vi "LS330_Main.vi"() -> ()   [LabVIEW 2021]
uses:
  Scale_Cont.ctl
  LS330_Message_Enum.ctl
  LS330_Status_Bundle.ctl
  LS330_LogSelector.ctl
  LS330_Setting_Cluster.ctl
panel:
  in  "Tab Control 4":enum32{"Overview", "History", "Actions"}(tab)
  out "Temp A":dbl caption="Temperature (K)" format="%.2g"
  out "Heater % A":dbl caption="Heater" format="%#_3g%%"
  out "Set Temp A":dbl caption="Current Set Temp (K)" format="%.2g"
  out "Ramp Rate A":dbl caption="Ramp Rate (K/min)" format="%.1g"
  out "Ramp Mode A":bool caption="Ramp Enabled"
  out "Ramp Busy A":bool caption="Ramp Busy"
  out "Heater Mode A":enum16{"Off", "Low", "Medium", "High"}(ring) caption="Heater Mode"
  out "Temp B":dbl caption="Temperature (K)" format="%.2g"
  out "Heater % B":dbl caption="Heater" format="%#_3g%%"
  out "Set Temp B":dbl caption="Current Set Temp (K)" format="%.2g"
  out "Ramp Rate B":dbl caption="Ramp Rate (K/min)" format="%.1g"
  out "Ramp Mode B":bool caption="Ramp Enabled"
  out "Ramp Busy B":bool caption="Ramp Busy"
  out "Heater Mode B":enum16{"Off", "Low", "Medium", "High"}(ring) caption="Heater Mode"
  out "Loop_A LED":bool
  out "Loop_B LED":bool
  out "Loop A Target":dbl caption="Target (K)" format="%.2g"
  out "Loop B Target":dbl caption="Target (K)" format="%.2g"
  in  "E-Stop":bool
  in  "Exit":bool
  out "XY Graph":T1(graph)
  in  "Tab Control 2":enum32{"Heater Options", "Options", "Read-Me!"}(tab)=enum."Read-Me!"
  in  "Tab Control 3":enum32{"Set Point Mode", "Ramp Mode"}(tab)
  in  "Set Temp A 2":dbl caption="Temp Set (K)" min=0.0 max=320.0 step=1.0 format="%.2g"
  in  "Set Range A":enum16{"Off", "Low", "Medium", "High"}(ring) caption="Range Set"
  in  "Set Temp B 2":dbl caption="Temp Set (K)" min=0.0 max=320.0 step=1.0 format="%.2g"
  in  "Set Range B":enum16{"Off", "Low", "Medium", "High"}(ring) caption="Range Set"
  in  "Read Settings":bool
  in  "Send Settings":bool
  in  "Read_A":bool
  in  "Send_A":bool
  in  "Rate_Temp_A":dbl caption="Ramp Rate (K/min)" min=0.0 max=100.0 step=0.1 format="%.1g"
  in  "End_Temp_A":dbl caption="Ramp End (K)" min=0.0 max=325.0 step=0.01 format="%.2g"
  in  "Start_Temp_A":dbl caption="Ramp Start (K)" min=0.0 max=325.0 step=0.01 format="%.2g"
  in  "Start_Temp_B":dbl caption="Ramp Start (K)" min=0.0 max=325.0 step=0.01 format="%.2g"
  in  "End_Temp_B":dbl caption="Ramp End (K)" min=0.0 max=325.0 step=0.01 format="%.2g"
  in  "Rate_Temp_B":dbl caption="Ramp Rate (K/min)" min=0.0 max=100.0 step=0.1 format="%.1g"
  in  "Send_B":bool
  in  "Read_B":bool
  in  "Set Range Ramp A":enum16{"Off", "Low", "Medium", "High"}(ring) caption="Range Set"
  in  "Set Range Ramp B":enum16{"Off", "Low", "Medium", "High"}(ring) caption="Range Set"
  in  "Tab Control":enum32{"Logging Options", "TC Options"}(tab)
  in  "Log Interval (seconds)":dbl=1.0
  in  "Save_Button":bool
  in  "Log File Location":path=path "C:/Users/C1Lab149/Documents/Labview/MDAQ_GUI_Prog/LS330_Main Folder/TempDir"
  in  "Clear_Button":bool
  in  "Chart Y-Axis Auto Scale":T2
  in  "Chart Interval (seconds)":dbl=1.0
  in  "Chart Zoom Width (hours)":dbl=1.0 min=0.01 max=24.0
  in  "Chart Time Width (hours)":dbl=12.0 min=0.01 max=42.0
  in  "Log File Name":string="LogFile_"
  in  "LakeShore VISA ID":refnum<visa-resource-name>="COM3"
  out "Error Panel":errorcluster
  out "HelpFile":string="8-March-22\n****** Read-Me file for LS335 Temperature Controller LabVIEW Program *******\n\nNotes:\n* LOG FILE SETTINGS:\nYou need to select the desired folder only, where you want the log files to be saved in. \nYou may also change the prefix of the saved files.\nThe file will be stored as prefixYYYY_MM_DD.txt (default is Log_YYYY_MM_DD.txt).\nDo this before starting the run.   \nIf you want to change the log settings during a run,\nstop the run, change the settings, and then restart the run.\n\n* AT STARTUP: if the program doesn't see the LS335, make sure that VISA ID is set to COM9 under the OPTIONS TAB.\n\n* FOR RAMPING: first set and achieve the initial temperature you want to start a ramp from.\n\tThen input the desired temperature you want to ramp to, set the ramp rate, and then enable the 'Toggle Ramping' slider before pressing the 'Send Settings' button.\n\tBoth the 'Ramp Enabled' and 'Ramp Busy' lights should be on and indicates that the LS335 is ramping to your desired temperature. NOTE: The 'Set Temp' indicator shows the steps towards the 'Target' temperature.\n\t\n\tOnce the 'Ramp' busy lights are off, the LS335 has finished the ramp procedure.\n\tYou may then either switch of the ramp slider which would revert the LS335 to the usual behaviour, or input a new set-point with the ramp slider still on. This will cause another ramp to occur.\n\n\tIf 'Send Settings' is pressed again with the 'Toggle Ramping' switch enabled, the ramp target is adjusted to the new value.\n\t\n\n"
  # "Loop A"
  # "Loop B"
  # "Heater A"
  # "Heater B"
  # "Heater A"
  # "Heater B"
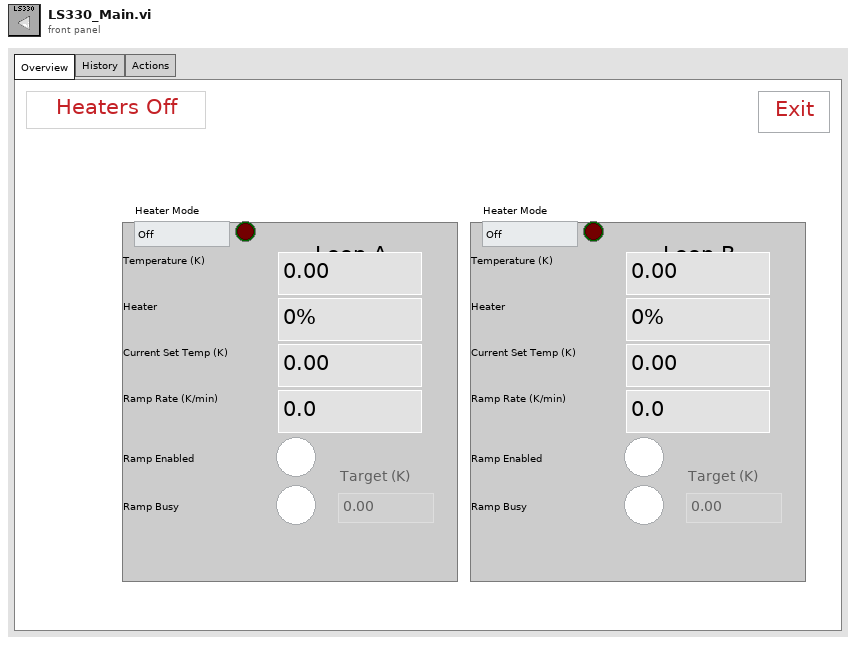
[diagram p1: front panel]
types:
  T1 = cluster{"Array":cluster{"time stamp":timestamp, "Numeric":dbl}[]}[]
  T2 = typedef "Scale_Cont.ctl" = enum16{"A & B", "A", "B"}
  T3 = typedef "LS330_LogSelector.ctl" = enum16{"NewFile", "Log", "OpenFile"}
  T4 = typedef "LS330_Status_Bundle.ctl" = cluster{"Temp":dbl, "Heater %":dbl, "Range":enum16{"Off", "Low", "Medium", "High"}, "Set Temp (K)":dbl, "Ramp Value":dbl, "Ramp Mode On/Off":bool, "Ramp Busy On/Off":bool}
  T5 = typedef "LS330_Message_Enum.ctl" = enum16{"Send Ramp B", "Send Ramp A", "Ramp Read Init B", "Ramp Read Init A", "Monitor TC", "Write Settings", "Read Settings", "E-Stop Write", "Quit Program"}
  T6 = cluster{cluster{timestamp, bool}, "Status IN":cluster{T4, T4}}
  T7 = cluster{"Array":cluster{"time stamp":timestamp, "Numeric":dbl}[], "Array":cluster{"time stamp":timestamp, "Numeric":dbl}[], "Array":cluster{"time stamp":timestamp, "Numeric":dbl}[], "Array":cluster{"time stamp":timestamp, "Numeric":dbl}[]}
  T8 = cluster{"Cluster":cluster{timestamp, "Checkbox":bool}, "Status IN":cluster{T4, T4}}
  T9 = cluster{"Array":cluster{timestamp, "Temp":dbl}[], "Array":cluster{timestamp, "Heater %":dbl}[], "Array":cluster{timestamp, "Temp":dbl}[], "Array":cluster{timestamp, "Heater %":dbl}[]}
  T10 = cluster{"Array":cluster{timestamp, "Heater %":dbl}[]}[]
  T11 = cluster{"TempA_Max":dbl, "TempA_Min":dbl, "HeaterA_Max":dbl, "HeaterA_Min":dbl, "TempB_Max":dbl, "TempB_Min":dbl, "HeaterB_Max":dbl, "HeaterB_Min":dbl}
  T12 = enum8{"Enabled", "Disabled", "Disabled and Grayed Out"}
  T13 = cluster{"seconds since 1Jan1904":timestamp, bool}
  T14 = cluster{cluster{"seconds since 1Jan1904":timestamp, bool}, "Status":cluster{T4, T4}}
  T15 = typedef "LS330_Setting_Cluster.ctl" = cluster{"Set Temp":dbl, "Set Range":enum16{"Off", "Low", "Medium", "High"}, "Set Ramp Rate":dbl, "Toggle Ramping":bool}
  T16 = cluster{"Setting Cluster":T15, "Setting Cluster":T15}
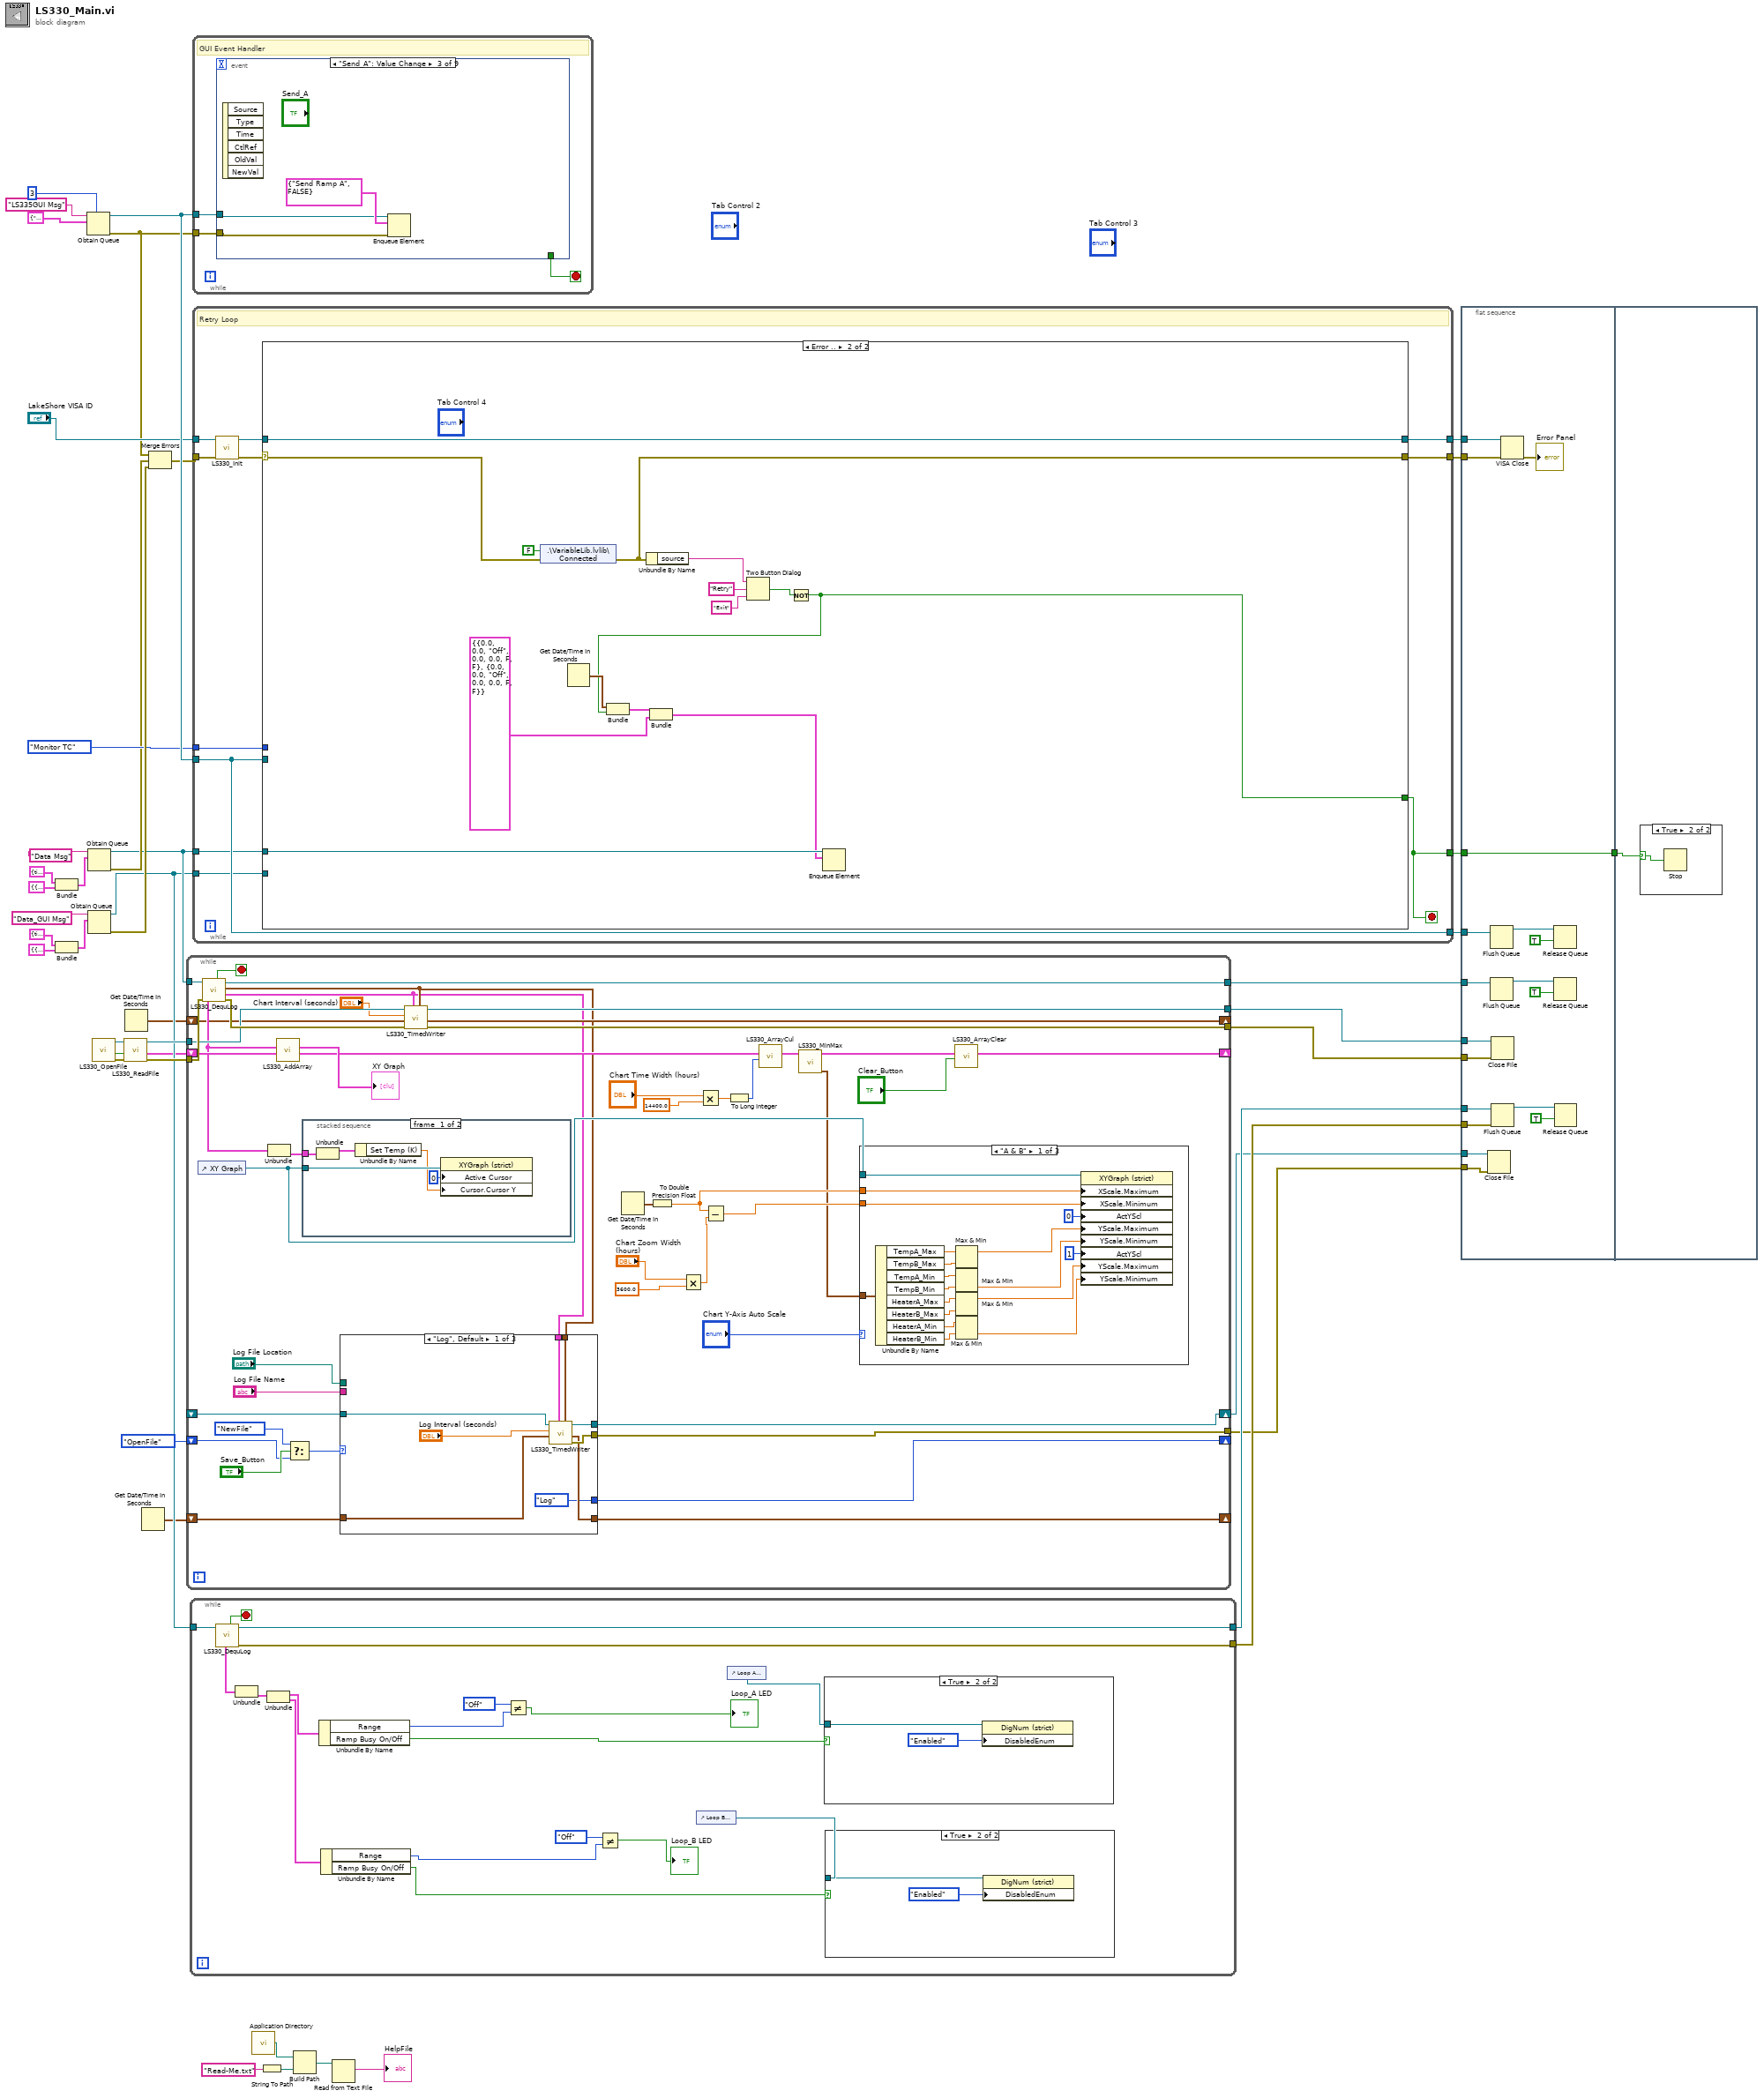
[diagram p0: block diagram]
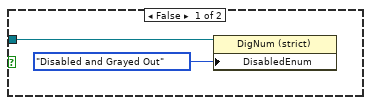
[diagram p2: hidden frame]
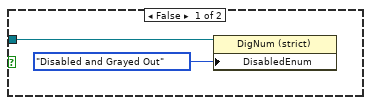
[diagram p3: hidden frame]
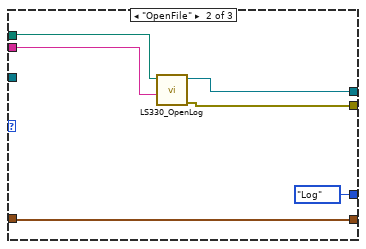
[diagram p4: hidden frame]
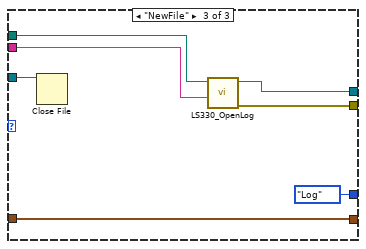
[diagram p5: hidden frame]
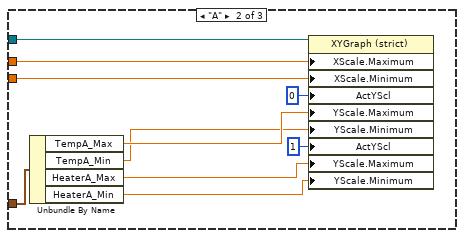
[diagram p6: hidden frame]
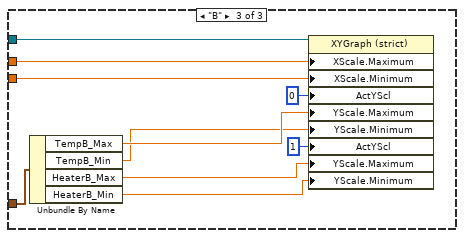
[diagram p7: hidden frame]
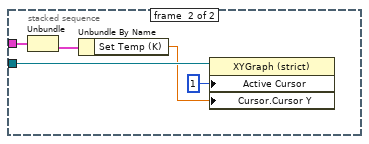
[diagram p8: hidden frame]
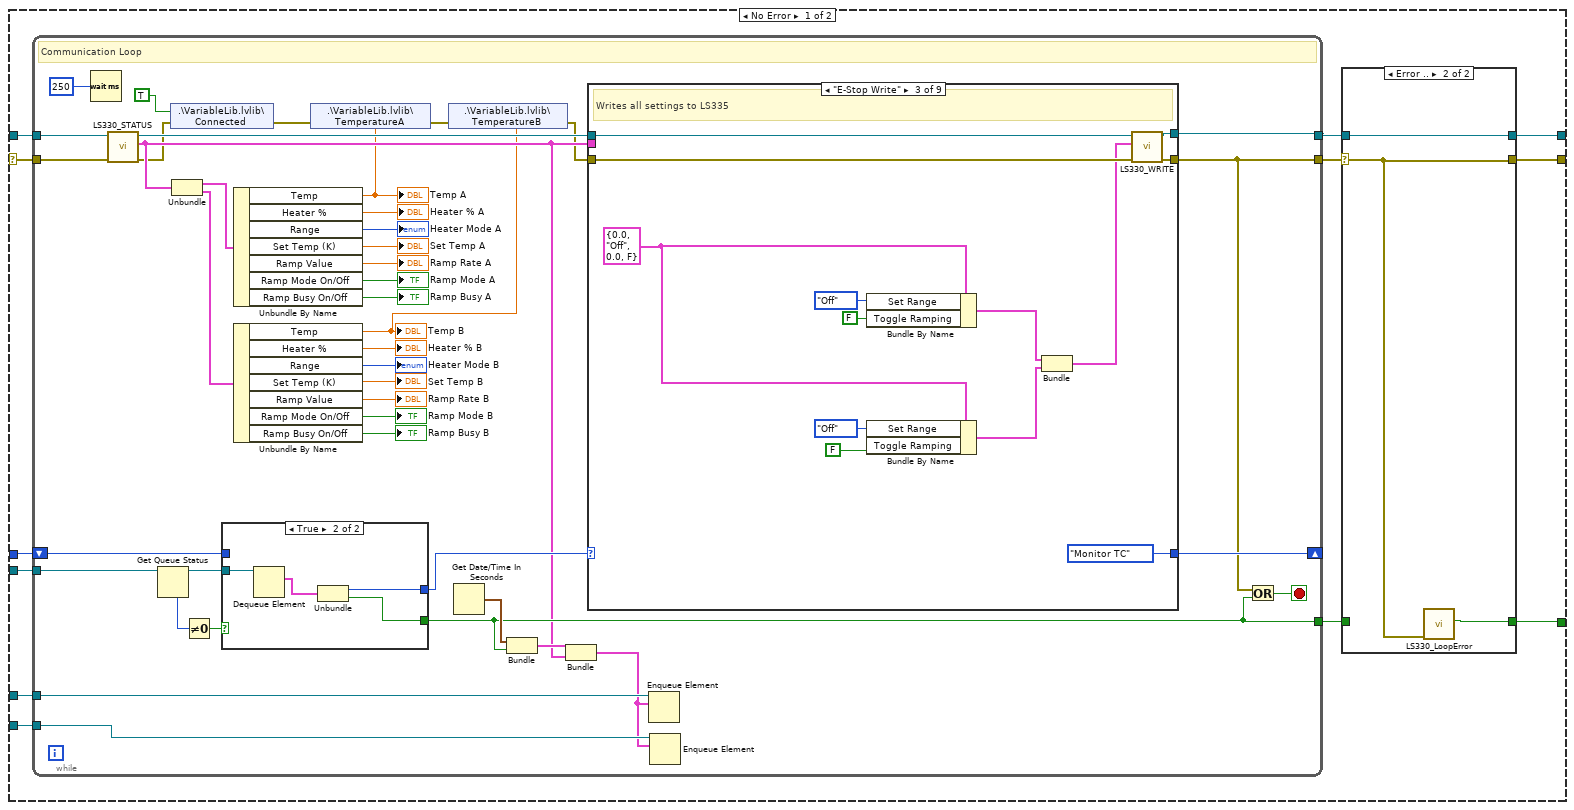
[diagram p10: hidden frame]
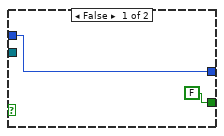
[diagram p12: hidden frame]
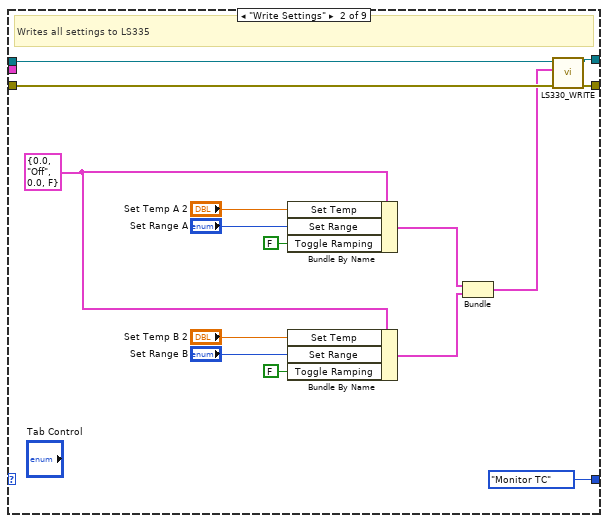
[diagram p14: hidden frame]
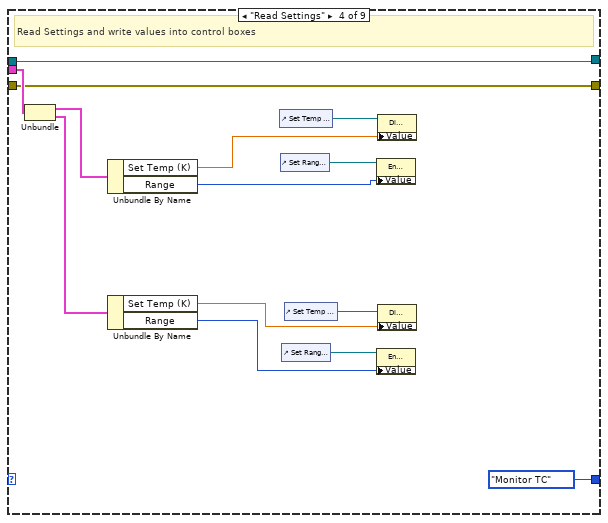
[diagram p15: hidden frame]
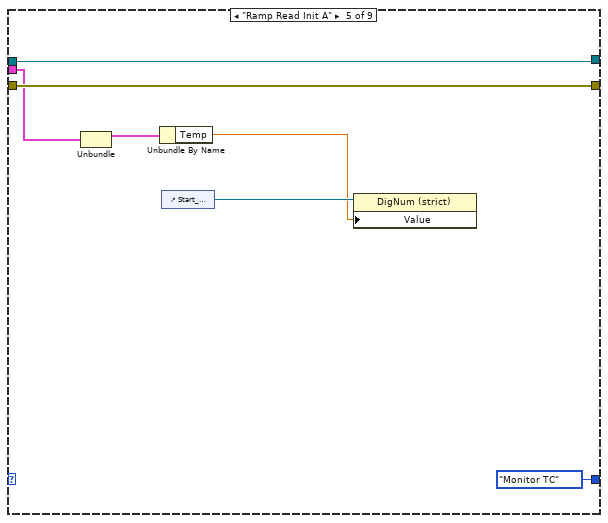
[diagram p16: hidden frame]
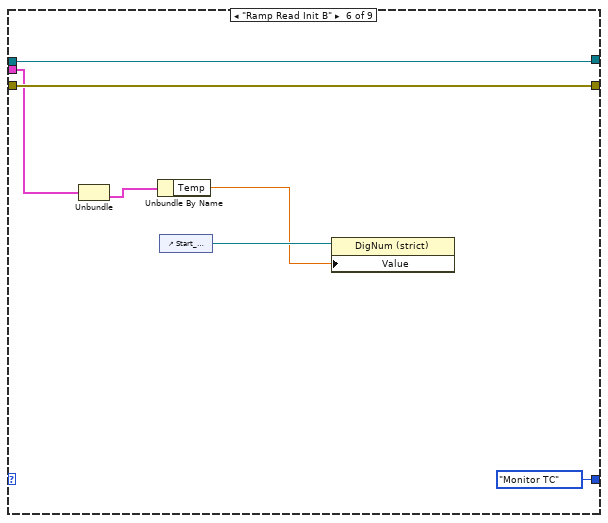
[diagram p17: hidden frame]
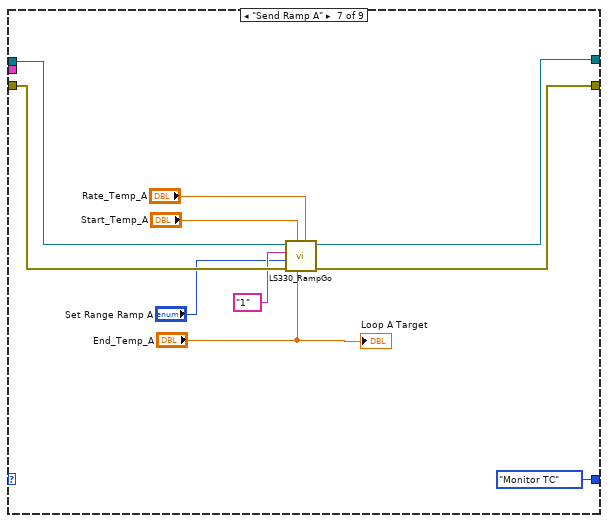
[diagram p18: hidden frame]
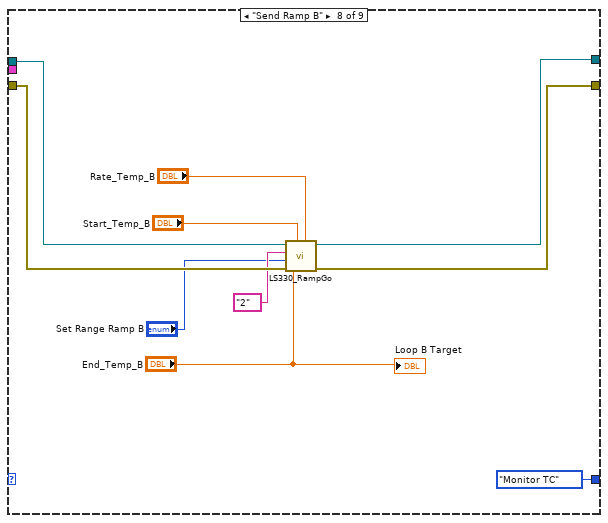
[diagram p19: hidden frame]
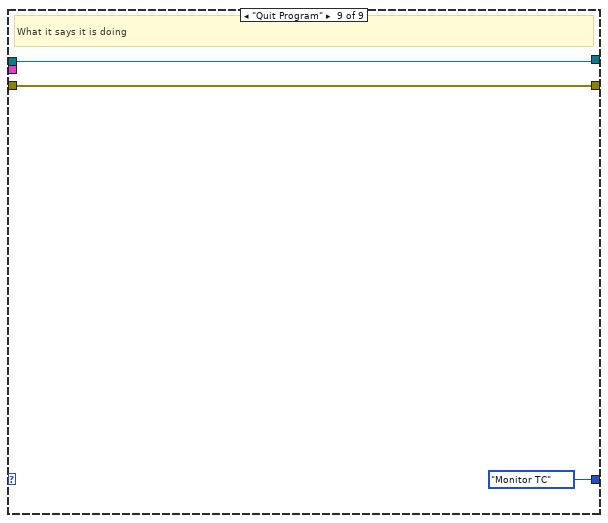
[diagram p20: hidden frame]
diagram:
  n1 = Bundle(cluster{timestamp, bool} {timestamp(0 s since 1904-01-01), FALSE}, "Status IN"=cluster{T4, T4} {{"Temp"=0.0, "Heater %"=0.0, "Range"=enum."Off", "Set Temp (K)"=0.0, "Ramp Value"=0.0, "Ramp Mode On/Off"=FALSE, "Ramp Busy On/Off"=FALSE}, {"Temp"=0.0, "Heater %"=0.0, "Range"=enum."Off", "Set Temp (K)"=0.0, "Ramp Value"=0.0, "Ramp Mode On/Off"=FALSE, "Ramp Busy On/Off"=FALSE}}) -> (w26:T6)  [unwired: 1 in]
  n2 = Bundle(cluster{timestamp, bool} {timestamp(0 s since 1904-01-01), FALSE}, "Status IN"=cluster{T4, T4} {{"Temp"=0.0, "Heater %"=0.0, "Range"=enum."Off", "Set Temp (K)"=0.0, "Ramp Value"=0.0, "Ramp Mode On/Off"=FALSE, "Ramp Busy On/Off"=FALSE}, {"Temp"=0.0, "Heater %"=0.0, "Range"=enum."Off", "Set Temp (K)"=0.0, "Ramp Value"=0.0, "Ramp Mode On/Off"=FALSE, "Ramp Busy On/Off"=FALSE}}) -> (w16:T6)  [unwired: 1 in]
  n3 = Obtain Queue(max queue size (-1, unlimited)=3, name (unnamed)="LS335GUI Msg", element data type=cluster{T5, bool} {enum."Monitor TC", TRUE}) -> (queue out=w45:refnum<queue>, error out=w32:errorcluster)  [unwired: 2 in, 1 out]
  n4 = Obtain Queue(name (unnamed)="Data Msg", element data type=w26) -> (queue out=w30:refnum<queue>, error out=w33:errorcluster)  [unwired: 3 in, 1 out]
  n5 = Obtain Queue(name (unnamed)="Data_GUI Msg", element data type=w16) -> (queue out=w21:refnum<queue>, error out=w46:errorcluster)  [unwired: 3 in, 1 out]
  n6 = call "LS330_OpenFile.vi"() -> ("error out"=w4:errorcluster, "file or folder exists?"=w5:bool, "File RefOut"=w6:refnum<file>)  [unwired: 9 in]
  n7 = call "LS330_ReadFile.vi"("error in"=w4, "File Exists?"=w5, "refnum"=w6) -> ("error out"=w28:errorcluster, "Cluster"=w20:T7, "refnum out"=w29:refnum<file>)  [unwired: 6 in]
  n8 = Get Date/Time In Seconds() -> (seconds since 1Jan1904=w19:timestamp)
  n9 = Get Date/Time In Seconds() -> (seconds since 1Jan1904=w3:timestamp)
  n10 = Merge Errors(w32, w33, w46) -> (w31:errorcluster)
  n11 = while {
    tunnel: w30 -> [w91]
    tunnel: w29 -> [w89]
    tunnel: w28 -> [w93]
    shift-right: [w62] -> _
    shift-left: w20 -> [w88]
    tunnel: [w90] -> w24
    tunnel: [w87] -> w23
    tunnel: [w86] -> w22
    shift-right: [w80] -> _
    shift-left: w19 -> [w81]
    shift-right: [w49] -> _
    shift-left: LS330_LogSelector."OpenFile" -> [w59]
    shift-right: [w51] -> _
    shift-left: w3 -> [w53]
    tunnel: [w52] -> w1
    shift-right: [w50] -> w2
    shift-left: _ -> [w56]
    stop <- w84 stop-if-true
    n12 = control-ref of="XY Graph"() -> (w78:refnum<vi>)
    n13 = call "LS330_DequLog.vi"("error in"=w93, "Queue in"=w91) -> ("error out"=w92:errorcluster, "Status Out"=w54:cluster{T4, T4}, "Time Stamp"=w55:timestamp, "Queue out"=w90:refnum<queue>, "Terminate?"=w84:bool, "Status/Time  Out"=w82:T8)  [unwired: 4 in]
    n14 = Unbundle(w82) -> ("Status IN"=w83:cluster{T4, T4})  [unwired: 1 out]
    n15 = call "LS330_AddArray.vi"("Array Cluster IN"=w88, "Queue IN"=w82) -> ("Array Cluster OUT"=w71:T9, "XY Plot Data"=→"XY Graph":T10)  [unwired: 8 in]
    n16 = Select(t=LS330_LogSelector."NewFile", s="Save_Button", f=w59) -> (s? t:f=w57:T3)
    n17 = stacked-sequence {
      tunnel: w78 -> [w158 w163]
      tunnel: w83 -> [w157 w162]
      frame #0 {
        n18 = Unbundle(w157) -> (w156:T4)  [unwired: 1 out]
        n19 = Unbundle By Name(w156) -> ("Set Temp (K)"=w155:dbl)
        n20 = property class="XYGraph (strict)"(reference=w158, "Active Cursor"=u32 0, "Cursor.Cursor Y"=w155) -> ()  [unwired: 1 in, 2 out]
      }
      frame #1 {
        n21 = Unbundle(w162) -> (w160:T4)  [unwired: 1 out]
        n22 = Unbundle By Name(w160) -> ("Set Temp (K)"=w161:dbl)
        n23 = property class="XYGraph (strict)"(reference=w163, "Active Cursor"=u32 1, "Cursor.Cursor Y"=w161) -> ()  [unwired: 1 in, 2 out]
      }
    }
    n24 = case shown="\"Log\", Default" w57 {
      tunnel: w56 -> [w94 _ w115]
      tunnel: w55 -> [w102 _ _]
      tunnel: w54 -> [w101 _ _]
      tunnel: w53 -> [w100 w105 w110]
      tunnel: [w99 w107 w111] -> w52
      tunnel: [w98 w105 w110] -> w51
      tunnel: [w97 w108 w112] -> w50
      tunnel: [LS330_LogSelector."Log" ("t") LS330_LogSelector."Log" ("t") LS330_LogSelector."Log" ("t")] -> w49
      tunnel: "Log File Name" -> [_ w104 w113]
      tunnel: "Log File Location" -> [_ w103 w114]
      frame "Log", Default {
        n25 = call "LS330_TimedWriter.vi"("Time Stamp"=w102, "Status In"=w101, "Time Check In"=w100, "Interval"="Log Interval (seconds)", "Byte Stream File in"=w94) -> ("error out"=w99:errorcluster, "Time Check Out"=w98:timestamp, "Byte Stream File out"=w97:refnum<file>)  [unwired: 4 in]
      }
      frame "OpenFile" {
        n26 = call "LS330_OpenLog.vi"("Prefix"=w104, "Log Location"=w103) -> ("error out"=w107:errorcluster, "File RefOut"=w108:refnum<file>)  [unwired: 7 in, 1 out]
      }
      frame "NewFile" {
        n27 = Close File(refnum=w115) -> ()  [unwired: 1 in, 2 out]
        n28 = call "LS330_OpenLog.vi"("Prefix"=w113, "Log Location"=w114) -> ("error out"=w111:errorcluster, "File RefOut"=w112:refnum<file>)  [unwired: 7 in, 1 out]
      }
    }
    n29 = call "LS330_TimedWriter.vi"("Time Stamp"=w55, "Status In"=w54, "error in (no error)"=w92, "Time Check In"=w81, "Interval"="Chart Interval (seconds)", "Byte Stream File in"=w89) -> ("error out"=w86:errorcluster, "Time Check Out"=w80:timestamp, "Byte Stream File out"=w87:refnum<file>)  [unwired: 3 in]
    n30 = Get Date/Time In Seconds() -> (seconds since 1Jan1904=w77:timestamp)
    n31 = To Double Precision Float(number=w77) -> (double precision float=w76:dbl)
    n32 = Multiply(x="Chart Zoom Width (hours)", y=3600.0) -> (x*y=w73:dbl)
    n33 = Multiply(x="Chart Time Width (hours)", y=14400.0) -> (x*y=w68:dbl)
    n34 = Subtract(x=w76, y=w73) -> (x-y=w72:dbl)
    n35 = To Long Integer(number=w68) -> (32bit integer=w67:i32)
    n36 = call "LS330_ArrayCul.vi"("Max Size"=w67, "Cluster Array IN"=w71) -> ("output cluster"=w66:T7)  [unwired: 9 in]
    n37 = call "LS330_MinMax.vi"("Input Cluster"=w66) -> ("Value Cluster"=w64:T11, "output cluster"=w63:T7)  [unwired: 9 in]
    n38 = case shown="\"A & B\"" "Chart Y-Axis Auto Scale" {
      tunnel: w78 -> [w133 w143 w153]
      tunnel: w76 -> [w132 w142 w152]
      tunnel: w72 -> [w131 w141 w151]
      tunnel: w64 -> [w130 w140 w150]
      frame "A & B" {
        n39 = Unbundle By Name(w130) -> ("TempA_Max"=w129:dbl, "TempB_Max"=w128:dbl, "TempA_Min"=w125:dbl, "TempB_Min"=w124:dbl, "HeaterA_Max"=w121:dbl, "HeaterB_Max"=w120:dbl, "HeaterA_Min"=w118:dbl, "HeaterB_Min"=w117:dbl)
        n40 = Max & Min(x=w129, y=w128) -> (max(x,y)=w126:dbl)  [unwired: 1 out]
        n41 = Max & Min(x=w125, y=w124) -> (min(x,y)=w123:dbl)  [unwired: 1 out]
        n42 = Max & Min(x=w121, y=w120) -> (max(x,y)=w119:dbl)  [unwired: 1 out]
        n43 = Max & Min(x=w118, y=w117) -> (min(x,y)=w116:dbl)  [unwired: 1 out]
        n44 = property class="XYGraph (strict)"(reference=w133, "XScale.Maximum"=w132, "XScale.Minimum"=w131, "ActYScl"=0 ("Active Y Scale"), "YScale.Maximum"=w126, "YScale.Minimum"=w123, "ActYScl"=1 ("Active Y Scale"), "YScale.Maximum"=w119, "YScale.Minimum"=w116) -> ()  [unwired: 1 in, 2 out]
      }
      frame "A" {
        n45 = Unbundle By Name(w140) -> ("TempA_Max"=w137:dbl, "TempA_Min"=w136:dbl, "HeaterA_Max"=w135:dbl, "HeaterA_Min"=w134:dbl)
        n46 = property class="XYGraph (strict)"(reference=w143, "XScale.Maximum"=w142, "XScale.Minimum"=w141, "ActYScl"=0 ("Active Y Scale"), "YScale.Maximum"=w137, "YScale.Minimum"=w136, "ActYScl"=1 ("Active Y Scale"), "YScale.Maximum"=w135, "YScale.Minimum"=w134) -> ()  [unwired: 1 in, 2 out]
      }
      frame "B" {
        n47 = Unbundle By Name(w150) -> ("TempB_Max"=w147:dbl, "TempB_Min"=w146:dbl, "HeaterB_Max"=w145:dbl, "HeaterB_Min"=w144:dbl)
        n48 = property class="XYGraph (strict)"(reference=w153, "XScale.Maximum"=w152, "XScale.Minimum"=w151, "ActYScl"=0 ("Active Y Scale"), "YScale.Maximum"=w147, "YScale.Minimum"=w146, "ActYScl"=1 ("Active Y Scale"), "YScale.Maximum"=w145, "YScale.Minimum"=w144) -> ()  [unwired: 1 in, 2 out]
      }
    }
    n49 = call "LS330_ArrayClear.vi"("Clear"="Clear_Button", "input cluster"=w63) -> ("output cluster"=w62:T7)  [unwired: 9 in]
  }
  n50 = while {
    tunnel: w21 -> [w181]
    tunnel: [w164] -> w14
    tunnel: [w179] -> w13
    stop <- w180 stop-if-true
    n51 = call "LS330_DequLog.vi"("Queue in"=w181) -> ("error out"=w179:errorcluster, "Queue out"=w164:refnum<queue>, "Terminate?"=w180:bool, "Status/Time  Out"=w178:T8)  [unwired: 5 in, 2 out]
    n52 = Unbundle(w178) -> ("Status IN"=w177:cluster{T4, T4})  [unwired: 1 out]
    n53 = Unbundle(w177) -> (w176:T4, w175:T4)
    n54 = Unbundle By Name(w176) -> ("Range"=w174:enum16{"Off", "Low", "Medium", "High"}, "Ramp Busy On/Off"=w168:bool)
    n55 = Unbundle By Name(w175) -> ("Range"=w170:enum16{"Off", "Low", "Medium", "High"}, "Ramp Busy On/Off"=w165:bool)
    n56 = Not Equal?(x=enum16{"Off", "Low", "Medium", "High"}."Off", y=w174) -> (x != y?=→"Loop_A LED":bool)
    n57 = Not Equal?(x=enum16{"Off", "Low", "Medium", "High"}."Off", y=w170) -> (x != y?=→"Loop_B LED":bool)
    n58 = control-ref of="Loop B Target"() -> (w166:refnum<vi>)
    n59 = control-ref of="Loop A Target"() -> (w167:refnum<vi>)
    n60 = case shown="True" w168 {
      tunnel: w167 -> [w187 w189]
      frame False {
        n61 = property class="DigNum (strict)"(reference=w187, "DisabledEnum"=T12."Disabled and Grayed Out" ("Disabled")) -> ()  [unwired: 1 in, 2 out]
      }
      frame True {
        n62 = property class="DigNum (strict)"(reference=w189, "DisabledEnum"=T12."Enabled" ("Disabled")) -> ()  [unwired: 1 in, 2 out]
      }
    }
    n63 = case shown="True" w165 {
      tunnel: w166 -> [w183 w185]
      frame False {
        n64 = property class="DigNum (strict)"(reference=w183, "DisabledEnum"=T12."Disabled and Grayed Out" ("Disabled")) -> ()  [unwired: 1 in, 2 out]
      }
      frame True {
        n65 = property class="DigNum (strict)"(reference=w185, "DisabledEnum"=T12."Enabled" ("Disabled")) -> ()  [unwired: 1 in, 2 out]
      }
    }
  }
  n66 = while "GUI Event Handler" {
    tunnel: w45 -> [w192]
    tunnel: w32 -> [w191]
    stop <- w190 stop-if-true
    # "GUI Event Handler"
    n67 = event shown="[2] \"Send_A\": Value Change" {
      selector: _ -> [_ _ _ _ _ _ _ _ _]
      dyn-events: _ -> [_ _ _ _ _ _ _ _ _]
      timeout: _ -> [_ _ _ _ _ _ _ _ _]
      tunnel: w192 -> [_ w195 w198 w201 w204 w207 w211 w216 w220]
      tunnel: w191 -> [_ w194 w197 w200 w203 w206 w209 w214 w219]
      tunnel: [_ FALSE _ _ _ _ FALSE TRUE FALSE] -> w190
      event Timeout {
        n68 = event-data() -> ()  [unwired: 1 in, 3 out]
      }
      event "Send Settings": Value Change {
        n69 = event-data() -> ()  [unwired: 1 in, 6 out]
        n70 = Enqueue Element(queue=w195, element=cluster{T5, bool} {enum."Write Settings", FALSE}, error in (no error)=w194) -> ()  [unwired: 1 in, 3 out]
      }
      event "Send_A": Value Change {
        n71 = event-data() -> ()  [unwired: 1 in, 6 out]
        n72 = Enqueue Element(queue=w198, element=cluster{T5, bool} {enum."Send Ramp A", FALSE}, error in (no error)=w197) -> ()  [unwired: 1 in, 3 out]
      }
      event "Send_B": Value Change {
        n73 = event-data() -> ()  [unwired: 1 in, 6 out]
        n74 = Enqueue Element(queue=w201, element=cluster{T5, bool} {enum."Send Ramp B", FALSE}, error in (no error)=w200) -> ()  [unwired: 1 in, 3 out]
      }
      event "Read_A": Value Change {
        n75 = event-data() -> ()  [unwired: 1 in, 6 out]
        n76 = Enqueue Element(queue=w204, element=cluster{T5, bool} {enum."Ramp Read Init A", FALSE}, error in (no error)=w203) -> ()  [unwired: 1 in, 3 out]
      }
      event "Read_B": Value Change {
        n77 = event-data() -> ()  [unwired: 1 in, 6 out]
        n78 = Enqueue Element(queue=w207, element=cluster{T5, bool} {enum."Ramp Read Init B", FALSE}, error in (no error)=w206) -> ()  [unwired: 1 in, 3 out]
      }
      event "Read Settings": Value Change {
        n79 = event-data() -> ()  [unwired: 1 in, 6 out]
        n80 = Enqueue Element(queue=w211, element=cluster{T5, bool} {enum."Read Settings", FALSE}, error in (no error)=w209) -> ()  [unwired: 1 in, 3 out]
      }
      event "Exit": Value Change {
        n81 = event-data() -> ()  [unwired: 1 in, 6 out]
        n82 = Enqueue Element At Opposite End(queue=w216, element=cluster{T5, bool} {enum."Monitor TC", TRUE}, error in (no error)=w214) -> ()  [unwired: 1 in, 3 out]
      }
      event "E-Stop": Value Change {
        n83 = event-data() -> ()  [unwired: 1 in, 6 out]
        n84 = Enqueue Element(queue=w220, element=cluster{T5, bool} {enum."E-Stop Write", FALSE}, error in (no error)=w219) -> ()  [unwired: 1 in, 3 out]
      }
    }
  }
  n85 = while {
    tunnel: w45 -> [w226]
    tunnel: LS330_Message_Enum."Monitor TC" -> [w228]
    tunnel: w31 -> [w227]
    tunnel: [w224] -> w38
    tunnel: "LakeShore VISA ID" -> [w231]
    tunnel: [w225] -> w39
    tunnel: [w226] -> w37
    tunnel: [w222] -> w35
    tunnel: w30 -> [w223]
    tunnel: w21 -> [w221]
    stop <- w222 stop-if-true
    # "Retry Loop"
    n86 = call "LS330_Init.vi"("error in"=w227, "VISA resource name"=w231) -> ("error out"=w230:errorcluster, "VISA resource name out"=w229:refnum<visa-resource-name>)  [unwired: 8 in]
    n87 = case shown="Error .." w230 {
      selector: w230 -> [w242 w382]
      tunnel: w229 -> [w243 w393]
      tunnel: w228 -> [w241 _]
      tunnel: w226 -> [w240 _]
      tunnel: [w236 w381] -> w224
      tunnel: [w237 w393] -> w225
      tunnel: [w233 w383] -> w222
      tunnel: w223 -> [w235 w388]
      tunnel: w221 -> [w232 _]
      frame No Error {
        n88 = while {
          tunnel: w243 -> [w291]
          tunnel: w242 -> [w290]
          tunnel: [w274] -> w239
          tunnel: [w266] -> w238
          shift-right: [w273] -> _
          shift-left: w241 -> [w268]
          tunnel: w240 -> [w272]
          tunnel: [w261] -> w234
          tunnel: w235 -> [w263]
          tunnel: w232 -> [w258]
          stop <- w265 stop-if-true
          # "Communication Loop"
          n89 = Wait (ms)(milliseconds to wait=u32 250) -> ()  [unwired: 1 out]
          n90 = call "LS330_STATUS.vi"("error in (no error)"=w290, "VISA Refnum in"=w291) -> ("error out"=w254:errorcluster, "Status"=w259:cluster{T4, T4}, "VISA resource name out"=w275:refnum<visa-resource-name>)  [unwired: 7 in]
          n91 = Get Queue Status(queue=w272) -> (queue out=w269:refnum<queue>, # elements in queue=w270:i32)  [unwired: 2 in, 6 out]
          n92 = shared-variable ".\\VariableLib.lvlib\\Connected"(TRUE ("Connected"), error in=w254) -> (error out=w253:errorcluster)
          n93 = Unbundle(w259) -> (w277:T4, w276:T4)
          n94 = Not Equal To 0?(x=w270) -> (x != 0?=w271:bool)
          n95 = case shown="True" w271 {
            tunnel: w269 -> [_ w297]
            tunnel: w268 -> [w293 _]
            tunnel: [w293 w295] -> w267
            tunnel: [FALSE w294] -> w261
            frame False {
            }
            frame True {
              n96 = Dequeue Element(queue=w297) -> (element=w296:cluster{T5, bool})  [unwired: 2 in, 3 out]
              n97 = Unbundle(w296) -> (w295:T5, w294:bool)
            }
          }
          n98 = Unbundle By Name(w277) -> ("Temp"=w255:dbl, "Heater %"=→"Heater % A":dbl, "Range"=→"Heater Mode A":enum16{"Off", "Low", "Medium", "High"}, "Set Temp (K)"=→"Set Temp A":dbl, "Ramp Value"=→"Ramp Rate A":dbl, "Ramp Mode On/Off"=→"Ramp Mode A":bool, "Ramp Busy On/Off"=→"Ramp Busy A":bool)
          "Temp A" <- w255
          n99 = Unbundle By Name(w276) -> ("Temp"=w250:dbl, "Heater %"=→"Heater % B":dbl, "Range"=→"Heater Mode B":enum16{"Off", "Low", "Medium", "High"}, "Set Temp (K)"=→"Set Temp B":dbl, "Ramp Value"=→"Ramp Rate B":dbl, "Ramp Mode On/Off"=→"Ramp Mode B":bool, "Ramp Busy On/Off"=→"Ramp Busy B":bool)
          "Temp B" <- w250
          n100 = shared-variable ".\\VariableLib.lvlib\\TemperatureA"(w255, error in=w253) -> (error out=w252:errorcluster)
          n101 = shared-variable ".\\VariableLib.lvlib\\TemperatureB"(w250, error in=w252) -> (error out=w251:errorcluster)
          n102 = Get Date/Time In Seconds() -> (seconds since 1Jan1904=w262:timestamp)
          n103 = Bundle("seconds since 1Jan1904"=w262, w261) -> (w260:T13)  [unwired: 1 in]
          n104 = Bundle(w260, "Status"=w259) -> (w257:T14)  [unwired: 1 in]
          n105 = case shown="\"E-Stop Write\"" w267 {
            selector: w267 -> [w298 _ _ _ _ _ _ _ _]
            tunnel: w275 -> [w300 w310 w325 w332 w348 w356 w366 w376 w378]
            tunnel: w251 -> [w299 w309 w324 w331 w347 w355 w365 w375 w377]
            tunnel: [w300 w307 w322 w332 w348 w356 w360 w373 w378] -> w274
            tunnel: [w299 w306 w321 w331 w347 w355 w359 w372 w377] -> w266
            tunnel: w259 -> [_ _ _ w340 w346 w354 _ _ _]
            tunnel: [w298 LS330_Message_Enum."Monitor TC" LS330_Message_Enum."Monitor TC" LS330_Message_Enum."Monitor TC" LS330_Message_Enum."Monitor TC" LS330_Message_Enum."Monitor TC" LS330_Message_Enum."Monitor TC" LS330_Message_Enum."Monitor TC" LS330_Message_Enum."Monitor TC"] -> w273
            frame "Monitor TC", Default {
              # "Pass through, does nothing"
            }
            frame "Write Settings" {
              w313 = T15 {"Set Temp"=0.0, "Set Range"=enum."Off", "Set Ramp Rate"=0.0, "Toggle Ramping"=FALSE} ("Setting Cluster")
              # "Writes all settings to LS335"
              n106 = Bundle By Name(cluster=w313, "Set Temp"="Set Temp A 2", "Set Range"="Set Range A", "Toggle Ramping"=FALSE) -> (w311:T15)
              n107 = Bundle By Name(cluster=w313, "Set Temp"="Set Temp B 2", "Set Range"="Set Range B", "Toggle Ramping"=FALSE) -> (w312:T15)
              n108 = Bundle("Setting Cluster"=w311, "Setting Cluster"=w312) -> (w308:T16)  [unwired: 1 in]
              n109 = call "LS330_WRITE.vi"("error in"=w309, "Input Cluster"=w308, "VISA resource name"=w310) -> ("error out"=w306:errorcluster, "VISA resource name out"=w307:refnum<visa-resource-name>)  [unwired: 7 in]
            }
            frame "E-Stop Write" {
              w328 = T15 {"Set Temp"=0.0, "Set Range"=enum."Off", "Set Ramp Rate"=0.0, "Toggle Ramping"=FALSE} ("Setting Cluster")
              # "Writes all settings to LS335"
              n110 = Bundle By Name(cluster=w328, "Set Range"=enum16{"Off", "Low", "Medium", "High"}."Off", "Toggle Ramping"=FALSE) -> (w326:T15)
              n111 = Bundle By Name(cluster=w328, "Set Range"=enum16{"Off", "Low", "Medium", "High"}."Off", "Toggle Ramping"=FALSE) -> (w327:T15)
              n112 = Bundle("Setting Cluster"=w326, "Setting Cluster"=w327) -> (w323:T16)  [unwired: 1 in]
              n113 = call "LS330_WRITE.vi"("error in"=w324, "Input Cluster"=w323, "VISA resource name"=w325) -> ("error out"=w321:errorcluster, "VISA resource name out"=w322:refnum<visa-resource-name>)  [unwired: 7 in]
            }
            frame "Read Settings" {
              # "Read Settings and write values into control boxes"
              n114 = Unbundle(w340) -> (w341:T4, w342:T4)
              n115 = Unbundle By Name(w341) -> ("Set Temp (K)"=w336:dbl, "Range"=w337:enum16{"Off", "Low", "Medium", "High"})
              n116 = Unbundle By Name(w342) -> ("Set Temp (K)"=w335:dbl, "Range"=w333:enum16{"Off", "Low", "Medium", "High"})
              n117 = control-ref of="Set Temp A 2"() -> (w339:refnum<vi>)
              n118 = control-ref of="Set Range A"() -> (w338:refnum<vi>)
              n119 = control-ref of="Set Range B"() -> (w334:refnum<vi>)
              n120 = control-ref of="Set Temp B 2"() -> (w329:refnum<vi>)
              n121 = property class="Enum (strict)"(reference=w338, "Value"=w337) -> ()  [unwired: 1 in, 2 out]
              n122 = property class="Enum (strict)"(reference=w334, "Value"=w333) -> ()  [unwired: 1 in, 2 out]
              n123 = property class="DigNum (strict)"(reference=w339, "Value"=w336) -> ()  [unwired: 1 in, 2 out]
              n124 = property class="DigNum (strict)"(reference=w329, "Value"=w335) -> ()  [unwired: 1 in, 2 out]
            }
            frame "Ramp Read Init A" {
              n125 = Unbundle(w346) -> (w345:T4)  [unwired: 1 out]
              n126 = Unbundle By Name(w345) -> ("Temp"=w343:dbl)
              n127 = control-ref of="Start_Temp_A"() -> (w344:refnum<vi>)
              n128 = property class="DigNum (strict)"(reference=w344, "Value"=w343) -> ()  [unwired: 1 in, 2 out]
            }
            frame "Ramp Read Init B" {
              n129 = Unbundle(w354) -> (w353:T4)  [unwired: 1 out]
              n130 = Unbundle By Name(w353) -> ("Temp"=w351:dbl)
              n131 = control-ref of="Start_Temp_B"() -> (w352:refnum<vi>)
              n132 = property class="DigNum (strict)"(reference=w352, "Value"=w351) -> ()  [unwired: 1 in, 2 out]
            }
            frame "Send Ramp A" {
              n133 = call "LS330_RampGo.vi"("Ramp Rate"="Rate_Temp_A", "Final Temp (K)"="End_Temp_A", "Initial Temp (K)"="Start_Temp_A", "error in"=w365, "Range"="Set Range Ramp A", "Heater"="1", "VISA resource name"=w366) -> ("error out"=w359:errorcluster, "VISA resource name out"=w360:refnum<visa-resource-name>)  [unwired: 3 in]
              "Loop A Target" <- "End_Temp_A"
            }
            frame "Send Ramp B" {
              n134 = call "LS330_RampGo.vi"("Ramp Rate"="Rate_Temp_B", "Final Temp (K)"="End_Temp_B", "Initial Temp (K)"="Start_Temp_B", "error in"=w375, "Range"="Set Range Ramp B", "Heater"="2", "VISA resource name"=w376) -> ("error out"=w372:errorcluster, "VISA resource name out"=w373:refnum<visa-resource-name>)  [unwired: 3 in]
              "Loop B Target" <- "End_Temp_B"
            }
            frame "Quit Program" {
              # "What it says it is doing"
            }
          }
          n135 = Enqueue Element(queue=w263, element=w257) -> ()  [unwired: 2 in, 3 out]
          n136 = Enqueue Element(queue=w258, element=w257) -> ()  [unwired: 2 in, 3 out]
          n137 = Or(x=w266, y=w261) -> (x .or. y?=w265:bool)
        }
        n138 = case shown="Error .." w238 {
          selector: w238 -> [w246 w248]
          tunnel: [w246 w248] -> w236
          tunnel: w239 -> [w245 w249]
          tunnel: [w245 w249] -> w237
          tunnel: [w244 w247] -> w233
          tunnel: w234 -> [w244 _]
          frame No Error {
          }
          frame Error {
            n139 = call "LS330_LoopError.vi"("error in"=w248) -> ("T button?"=w247:bool)  [unwired: 10 in]
          }
        }
      }
      frame Error {
        n140 = shared-variable ".\\VariableLib.lvlib\\Connected"(FALSE ("Connected"), error in=w382) -> (error out=w381:errorcluster)
        n141 = Get Date/Time In Seconds() -> (seconds since 1Jan1904=w387:timestamp)
        n142 = Unbundle By Name(w381) -> ("source"=w392:string)
        n143 = Two Button Dialog(message=w392, 1:"Exit" ("F button name (\"Cancel\")"), 2:"Retry" ("T button name (\"OK\")")) -> (T button?=w391:bool)
        n144 = Not(x=w391) -> (.not. x?=w383:bool)
        n145 = Bundle("seconds since 1Jan1904"=w387, w383) -> (w386:T13)  [unwired: 1 in]
        n146 = Bundle(w386, "Status"=cluster{T4, T4} {{"Temp"=0.0, "Heater %"=0.0, "Range"=enum."Off", "Set Temp (K)"=0.0, "Ramp Value"=0.0, "Ramp Mode On/Off"=FALSE, "Ramp Busy On/Off"=FALSE}, {"Temp"=0.0, "Heater %"=0.0, "Range"=enum."Off", "Set Temp (K)"=0.0, "Ramp Value"=0.0, "Ramp Mode On/Off"=FALSE, "Ramp Busy On/Off"=FALSE}}) -> (w385:T14)  [unwired: 1 in]
        n147 = Enqueue Element(queue=w388, element=w385) -> ()  [unwired: 2 in, 3 out]
      }
    }
  }
  n148 = call <vilib>:"Application Directory.vi"() -> ("Application Directory"=w12:path)
  n149 = String To Path(string="Read-Me.txt") -> (path=w10:path)
  n150 = Build Path(base path=w12, name or relative path=w10) -> (appended path=w9:path)
  n151 = Read from Text File(file (use dialog)=w9) -> (text=→"HelpFile":string)  [unwired: 3 in, 3 out]
  n152 = flat-sequence {
    tunnel: w39 -> [w410]
    tunnel: w38 -> [w409]
    tunnel: w37 -> [w406]
    tunnel: [w405] -> w36
    tunnel: w35 -> [w405]
    tunnel: w24 -> [w400]
    tunnel: w23 -> [w404]
    tunnel: w22 -> [w403]
    tunnel: w14 -> [w397]
    tunnel: w13 -> [w396]
    tunnel: w2 -> [w395]
    tunnel: w1 -> [w394]
    tunnel: w36 -> [w412]
    frame #0 {
      n153 = Close File(refnum=w395, error in=w394) -> ()  [unwired: 2 out]
      n154 = Flush Queue(queue=w406) -> (queue out=w408:refnum<queue>)  [unwired: 1 in, 2 out]
      n155 = Flush Queue(queue=w400) -> (queue out=w402:refnum<queue>)  [unwired: 1 in, 2 out]
      n156 = Close File(refnum=w404, error in=w403) -> ()  [unwired: 2 out]
      n157 = Flush Queue(queue=w397, error in (no error)=w396) -> (queue out=w399:refnum<queue>)  [unwired: 2 out]
      n158 = VISA Close(VISA resource name=w410, error in (no error)=w409) -> (error out=→"Error Panel":errorcluster)
      n159 = Release Queue(queue=w408, force destroy? (F)=TRUE) -> ()  [unwired: 1 in, 3 out]
      n160 = Release Queue(queue=w402, force destroy? (F)=TRUE) -> ()  [unwired: 1 in, 3 out]
      n161 = Release Queue(queue=w399, force destroy? (F)=TRUE) -> ()  [unwired: 1 in, 3 out]
    }
    frame #1 {
      n162 = case shown="True" w412 {
        selector: w412 -> [_ w413]
        frame False {
        }
        frame True {
          n163 = Stop(stop? (T)=w413) -> ()
        }
      }
    }
  }
